vi "h.DETECTION.GetAvailableDetectionSettings.vi"(8 "error in":errorcluster, 11 "Connection ID":refnum<k5>) -> (0 "error out":errorcluster, 2 "Instrument Detection Settings":T1[](array[typedef]), 3 "Connection ID out":refnum<k5>)   [LabVIEW 2016, in "h.Library.lvlib"]
uses:
  h.Library.lvlib
  h.DETECTION.PeakDetectionPreset.ctl
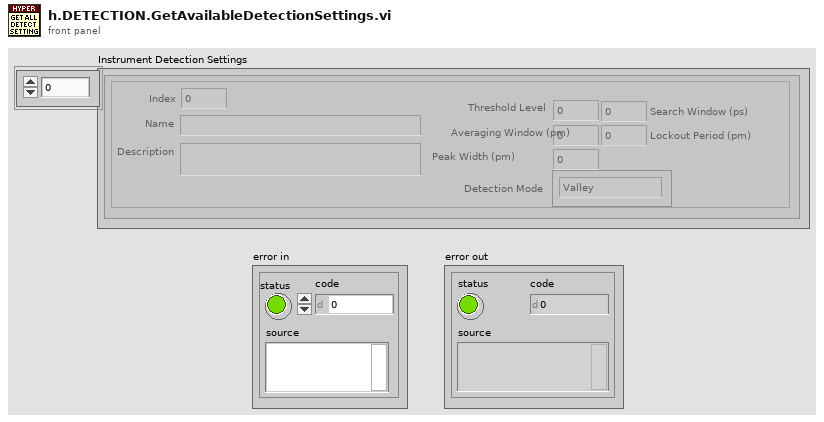
[diagram p1: front panel]
types:
  T1 = typedef "h.Library.lvlib/h.DETECTION.PeakDetectionPreset.ctl" = cluster{"Index":u8, "Name":string, "Description":string, "Detection Mode":enum32{"Valley", "Peak"}, "Averaging Window (pm)":i32, "Peak Width (pm)":i32, "Lockout Period (pm)":i32, "Search Window (ps)":i32, "Threshold Level":i32}
  T2 = enum16{"big-endian, network order", "native, host order", "little-endian"}
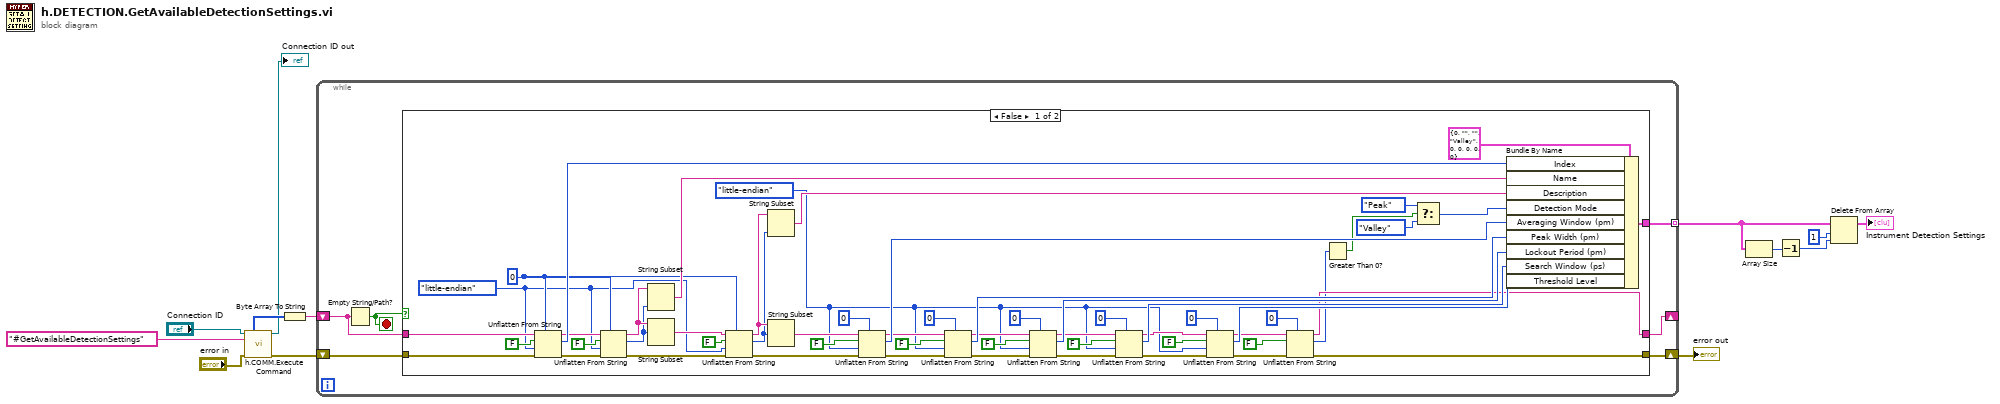
[diagram p0: block diagram]
diagram:
  n1 = call "h.COMM.Execute Command.vi"("Connection ID"="Connection ID", "Command"="#GetAvailableDetectionSettings", "error in"="error in") -> ("Content"=w11:u8[], "Connection ID out"=→"Connection ID out":refnum<k5>, "error out"=w3:errorcluster)  [unwired: 5 in, 5 out]
  n2 = Byte Array To String(unsigned byte array=w11) -> (string=w10:string)
  n3 = while {
    tunnel: [w17] -> w5 mode=indexing
    shift-right: [w16] -> _
    shift-left: w10 -> [w19]
    shift-right: [w15] -> w2
    shift-left: w3 -> [w14]
    stop <- w18 stop-if-true
    n4 = Empty String/Path?(string/path=w19) -> (empty?=w18:bool)
    n5 = case shown="False" w18 {
      tunnel: w19 -> [w76 w78]
      tunnel: w14 -> [w75 w77]
      tunnel: [w32 _] -> w17
      tunnel: [w27 w78] -> w16
      tunnel: [w26 w77] -> w15
      frame False {
        w20 = T2."little-endian" ("byte order (0:big-endian, network order)")
        w63 = u8 0
        w61 = T2."little-endian" ("byte order (0:big-endian, network order)")
        n6 = Unflatten From String(type=w63, binary string=w76, data includes array or string size? (T)=FALSE, byte order (0:big-endian, network order)=w61, error in (no error)=w75) -> (rest of the binary string=w70:string, value=w72:u8, error out=w69:errorcluster)
        n7 = Unflatten From String(type=w63, binary string=w70, data includes array or string size? (T)=FALSE, byte order (0:big-endian, network order)=w61, error in (no error)=w69) -> (rest of the binary string=w67:string, value=w66:u8, error out=w64:errorcluster)
        n8 = String Subset(string=w67, length (rest)=w66) -> (substring=w68:string)  [unwired: 1 in]
        n9 = String Subset(string=w67, offset (0)=w66) -> (substring=w62:string)  [unwired: 1 in]
        n10 = Unflatten From String(type=w63, binary string=w62, data includes array or string size? (T)=FALSE, byte order (0:big-endian, network order)=w61, error in (no error)=w64) -> (rest of the binary string=w59:string, value=w58:u8, error out=w55:errorcluster)
        n11 = String Subset(string=w59, length (rest)=w58) -> (substring=w60:string)  [unwired: 1 in]
        n12 = String Subset(string=w59, offset (0)=w58) -> (substring=w56:string)  [unwired: 1 in]
        n13 = Unflatten From String(type=u16 0, binary string=w56, data includes array or string size? (T)=FALSE, byte order (0:big-endian, network order)=w20, error in (no error)=w55) -> (rest of the binary string=w50:string, value=w53:u16, error out=w49:errorcluster)
        n14 = Unflatten From String(type=u16 0, binary string=w50, data includes array or string size? (T)=FALSE, byte order (0:big-endian, network order)=w20, error in (no error)=w49) -> (rest of the binary string=w45:string, value=w48:u16, error out=w44:errorcluster)
        n15 = Unflatten From String(type=u16 0, binary string=w45, data includes array or string size? (T)=FALSE, byte order (0:big-endian, network order)=w20, error in (no error)=w44) -> (rest of the binary string=w39:string, value=w43:u16, error out=w40:errorcluster)
        n16 = Unflatten From String(type=u16 0, binary string=w39, data includes array or string size? (T)=FALSE, byte order (0:big-endian, network order)=w20, error in (no error)=w40) -> (rest of the binary string=w34:string, value=w38:u16, error out=w35:errorcluster)
        n17 = Unflatten From String(type=0, binary string=w34, data includes array or string size? (T)=FALSE, byte order (0:big-endian, network order)=w20, error in (no error)=w35) -> (rest of the binary string=w29:string, value=w33:i32, error out=w28:errorcluster)
        n18 = Unflatten From String(type=u8 0, binary string=w29, data includes array or string size? (T)=FALSE, error in (no error)=w28) -> (rest of the binary string=w27:string, value=w24:u8, error out=w26:errorcluster)  [unwired: 1 in]
        n19 = Greater Than 0?(x=w24) -> (x > 0?=w25:bool)
        n20 = Select(t=enum32{"Valley", "Peak"}."Peak" ("Detection Mode"), s=w25, f=enum32{"Valley", "Peak"}."Valley" ("Detection Mode")) -> (s? t:f=w21:enum32{"Valley", "Peak"})
        n21 = Bundle By Name(cluster=T1 {"Index"=0, "Name"="", "Description"="", "Detection Mode"=enum."Valley", "Averaging Window (pm)"=0, "Peak Width (pm)"=0, "Lockout Period (pm)"=0, "Search Window (ps)"=0, "Threshold Level"=0} ("Preset"), "Index"=w72, "Name"=w68, "Description"=w60, "Detection Mode"=w21, "Averaging Window (pm)"=w53, "Peak Width (pm)"=w48, "Lockout Period (pm)"=w43, "Search Window (ps)"=w38, "Threshold Level"=w33) -> (w32:T1)
      }
      frame True {
      }
    }
  }
  "error out" <- w2
  n22 = Array Size(array=w5) -> (size(s)=w8:i32)
  n23 = Decrement(x=w8) -> (x-1=w7:i32)
  n24 = Delete From Array(array=w5, length=1, index=w7) -> (array with subset deleted=→"Instrument Detection Settings":T1[])  [unwired: 1 out]
